vi "lv-ros-bridge_read.vi"(8 "error in (no error)":errorcluster, 9 "subscribe message":string="{ \"op\": \"subscribe\", \"topic\" : \"/chatter_joy\" }", 10 "rosbridge port":u16=9090, 11 "rosbridge server IP":string="192.168.5.103") -> (0 "error out":errorcluster, 2 "axes":sgl[](array[numeric]), 3 "buttons":i32[](array[numeric]))   [LabVIEW 2013]
uses:
  <vilib>/Intelligent Energy/WebSockets API/WebSockets/WebSockets.lvlib
panel:
  out "incomming\nmessage":T1
  out "value":T1
  in  "?":T1
  out "raw frame":string
  in  "stop":bool
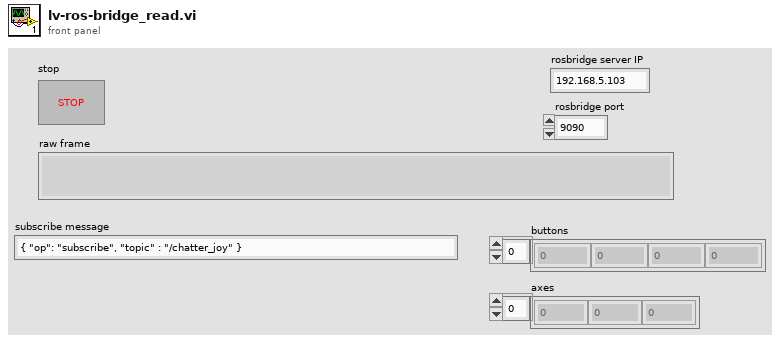
[diagram p1: front panel]
types:
  T1 = cluster{"topic":string, "msg":cluster{"header":cluster{"seq":u32, "stamp":cluster{"secs":u32, "nsecs":i32}, "frame_id":string}, "buttons":i32[], "axes":sgl[]}, "op":string}
  T2 = cluster{"header":cluster{"seq":u32, "stamp":cluster{"secs":u32, "nsecs":i32}, "frame_id":string}, "buttons":i32[], "axes":sgl[]}
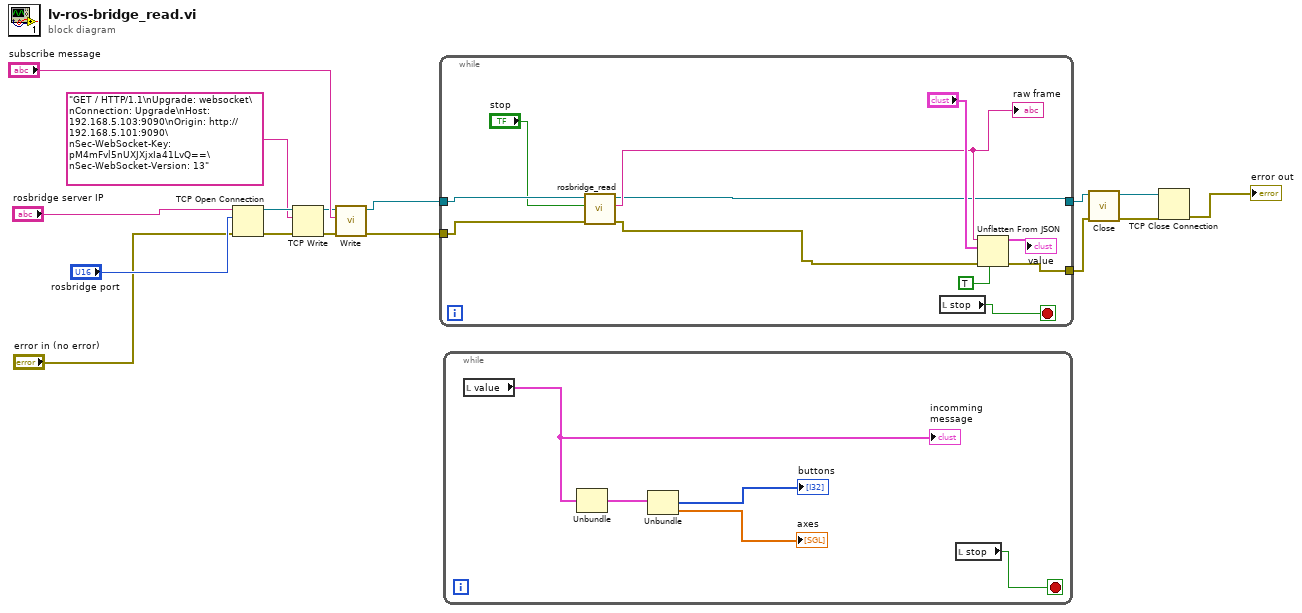
[diagram p0: block diagram]
diagram:
  n1 = TCP Open Connection(address="rosbridge server IP", remote port or service name="rosbridge port", error in (no error)="error in (no error)") -> (connection ID=w14:refnum<k5>, error out=w12:errorcluster)  [unwired: 2 in]
  n2 = TCP Write(connection ID=w14, data in="GET / HTTP/1.1\nUpgrade: websocket\nConnection: Upgrade\nHost: 192.168.5.103:9090\nOrigin: http://192.168.5.101:9090\nSec-WebSocket-Key: pM4mFvl5nUXJXjxIa41LvQ==\nSec-WebSocket-Version: 13", error in (no error)=w12) -> (connection ID out=w8:refnum<k5>, error out=w7:errorcluster)  [unwired: 1 in, 1 out]
  n3 = call <vilib>:"Write.vi"("error in (no error)"=w7, "Data"="subscribe message", "WebSocket Connection in"=w8) -> ("error out"=w1:errorcluster, "WebSocket Connection out"=w2:refnum<k5>)  [unwired: 7 in]
  n4 = while {
    tunnel: [w17] -> w6
    tunnel: [w27] -> w5
    tunnel: w2 -> [w22]
    tunnel: w1 -> [w19]
    stop <- w23 stop-if-true
    n5 = call "rosbridge_read.vi"("error in (no error)"=w19, "stop"="stop", "TCP Network Connection in"=w22) -> ("error out"=w18:errorcluster, "String"=w20:string, "TCP Network Connection out"=w17:refnum<k5>)  [unwired: 6 in]
    "raw frame" <- w20
    n6 = local read "stop"() -> (w23:bool)
    n7 = Unflatten From JSON(JSON string=w20, type and defaults="?", default null elements? (F)=TRUE, error in (no error)=w18) -> (value=→"value":T1, error out=w27:errorcluster)  [unwired: 3 in]
  }
  n8 = while {
    stop <- w28 stop-if-true
    n9 = local read "value"() -> (w32:T1)
    "incomming\nmessage" <- w32
    n10 = Unbundle(w32) -> ("msg"=w31:T2)  [unwired: 2 out]
    n11 = Unbundle(w31) -> ("buttons"=→"buttons":i32[], "axes"=→"axes":sgl[])  [unwired: 1 out]
    n12 = local read "stop"() -> (w28:bool)
  }
  n13 = call <vilib>:"Close.vi"("error in (no error)"=w5, "WebSocket Connection in"=w6) -> ("error out"=w9:errorcluster, "WebSocket Connection in"=w10:refnum<k5>)  [unwired: 8 in]
  n14 = TCP Close Connection(connection ID=w10, error in (no error)=w9) -> (error out=→"error out":errorcluster)  [unwired: 1 in, 1 out]
